vi "connect_key.vi"(8 "error in (no error)":errorcluster, 9 "Connection Name":string, 10 "Private_Public Key":T2, 11 "Connection Info.":T1={"Remote"="", "Username"="", "Port (22)"=22}) -> (0 "error out":errorcluster, 2 "isSshConnected":bool, 3 "Return String":string)   [LabVIEW 2022 SP3, in "LabSSH.lvlib"]
doc: "<License>This software is distributed under the BSD 3-Clause License. For the full license please see license.txt or visit www.labvolution.com/license</License>"
uses:
  LabSSH.lvlib
  Private Public Key..cluster.ctl
  Connection Info..cluster.ctl
  FGV State..enum.ctl
  D:/project/tvtEye/guard_tvt/tools/LabSSH Library/References/LabSSH.dll
  References/LabSSH.dll
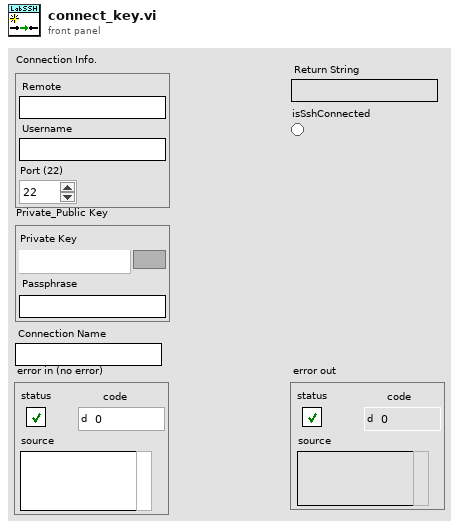
[diagram p1: front panel]
types:
  T1 = typedef "LabSSH.lvlib/Connection Info..cluster.ctl" = cluster{"Remote":string, "Username":string, "Port (22)":i32}
  T2 = typedef "LabSSH.lvlib/Private Public Key..cluster.ctl" = cluster{"Private Key":path, "Passphrase":string}
  T3 = typedef "LabSSH.lvlib/FGV State..enum.ctl" = enum16{"GET", "SET"}
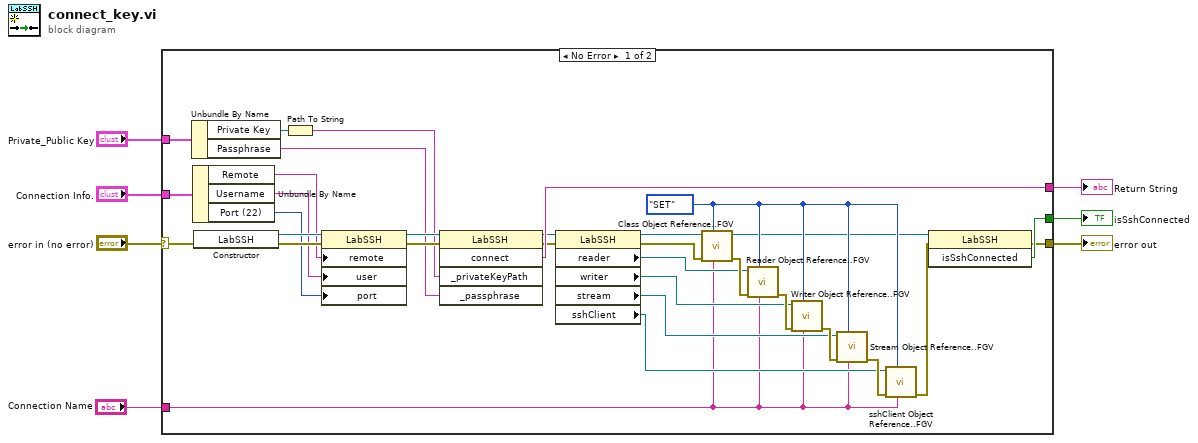
[diagram p0: block diagram]
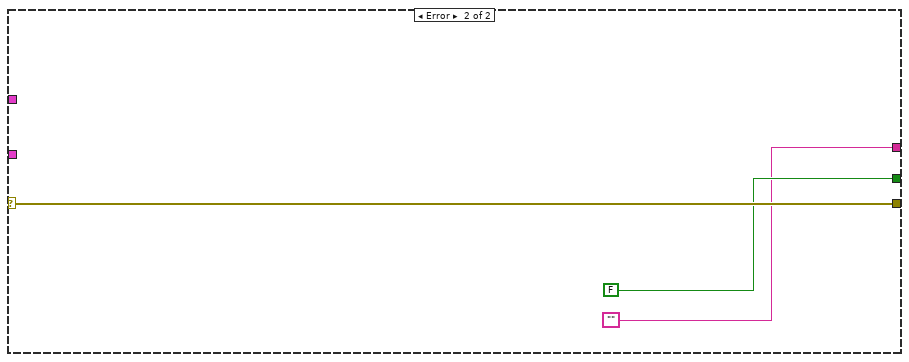
[diagram p2: hidden frame]
diagram:
  n1 = case shown="No Error" "error in (no error)" {
    selector: "error in (no error)" -> [w25 w42]
    tunnel: "Private_Public Key" -> [w35 _]
    tunnel: "Connection Info." -> [w34 _]
    tunnel: [w33 ""] -> w5
    tunnel: [w32 FALSE ("isSshConnected")] -> w4
    tunnel: [w24 w42] -> w3
    tunnel: "Connection Name" -> [w8 _]
    frame No Error {
      w13 = FGV_State..enum."SET" ("FGV State")
      n2 = Unbundle By Name(w35) -> ("Private Key"=w28:path, "Passphrase"=w26:string)
      n3 = Unbundle By Name(w34) -> ("Remote"=w31:string, "Username"=w30:string, "Port (22)"=w29:i32)
      n4 = constructor class="LabSSH" ("Constructor Node")(error in=w25) -> (reference out=w39:refnum<k24>, error out=w36:errorcluster)  [unwired: 2 in, 1 out]
      n5 = Path To String(path=w28) -> (string=w27:string)
      n6 = property on="Property Node" class="LabSSH"(reference=w39, error in=w36, "remote"=w31, "user"=w30, "port"=w29) -> (reference out=w38:refnum<k24>, error out=w37:errorcluster)
      n7 = invoke on="Invoke Node" class="LabSSH" method="connect"(reference=w38, error in=w37, "_privateKeyPath"=w27, "_passphrase"=w26) -> (reference out=w12:refnum<k24>, error out=w11:errorcluster, "connect"=w33:string)  [unwired: 1 in, 2 out]
      n8 = property class="LabSSH"(reference=w12, error in=w11) -> (reference out=w23:refnum<k24>, error out=w22:errorcluster, "reader"=w17:refnum<k24>, "writer"=w16:refnum<k24>, "stream"=w15:refnum<k24>, "sshClient"=w14:refnum<k24>)
      n9 = call "Class Object Reference..FGV.vi"("Connection Name"=w8, "FGV State (GET)"=w13, "error in (no error)"=w22, "LabSSH ref in"=w23) -> ("error out"=w21:errorcluster, "LabSSH ref out"=w10:refnum<k24>)  [unwired: 6 in]
      n10 = call "Reader Object Reference..FGV.vi"("Connection Name"=w8, "FGV State (GET)"=w13, "error in (no error)"=w21, "Reader ref in"=w17) -> ("error out"=w20:errorcluster)  [unwired: 6 in, 1 out]
      n11 = call "Writer Object Reference..FGV.vi"("Connection Name"=w8, "FGV State (GET)"=w13, "error in (no error)"=w20, "Writer ref in"=w16) -> ("error out"=w19:errorcluster)  [unwired: 6 in, 1 out]
      n12 = call "Stream Object Reference..FGV.vi"("Connection Name"=w8, "FGV State (GET)"=w13, "error in (no error)"=w19, "Stream ref in"=w15) -> ("error out"=w18:errorcluster)  [unwired: 6 in, 1 out]
      n13 = call "sshClient Object Reference..FGV.vi"("Connection Name"=w8, "FGV State (GET)"=w13, "error in (no error)"=w18, "sshClient ref in"=w14) -> ("error out"=w9:errorcluster)  [unwired: 6 in, 1 out]
      n14 = invoke on="Invoke Node" class="LabSSH" method="isSshConnected"(reference=w10, error in=w9) -> (error out=w24:errorcluster, "isSshConnected"=w32:bool)  [unwired: 1 in, 1 out]
    }
    frame Error {
    }
  }
  "error out" <- w3
  "isSshConnected" <- w4
  "Return String" <- w5
